vi "Goal Cases.vi"(3 "InArray":dbl[][](array[numeric])) -> (0 "Classification Error":bool, 1 "OutArray":dbl[][](array[numeric]))   [LabVIEW 2012]
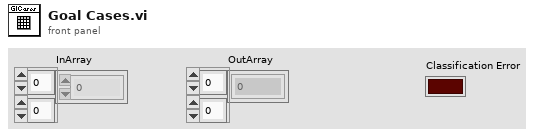
[diagram p1: front panel]
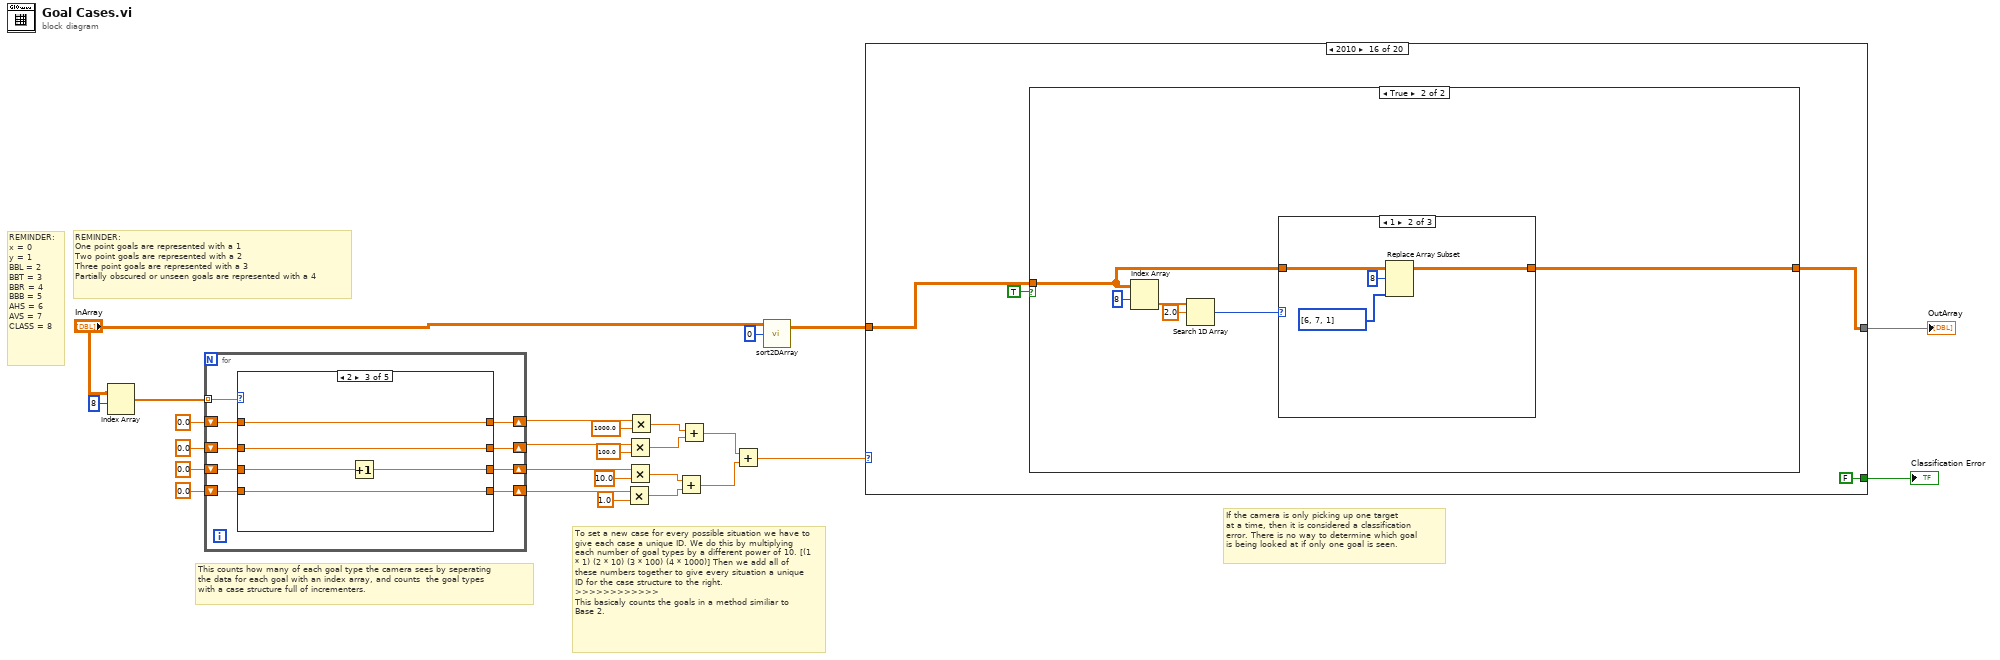
[diagram p0: block diagram]
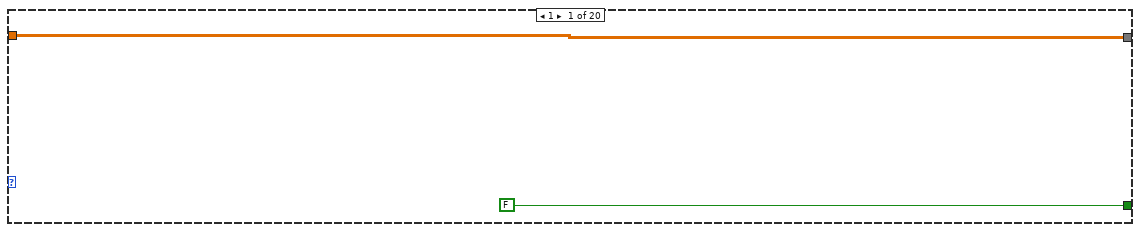
[diagram p2: hidden frame]
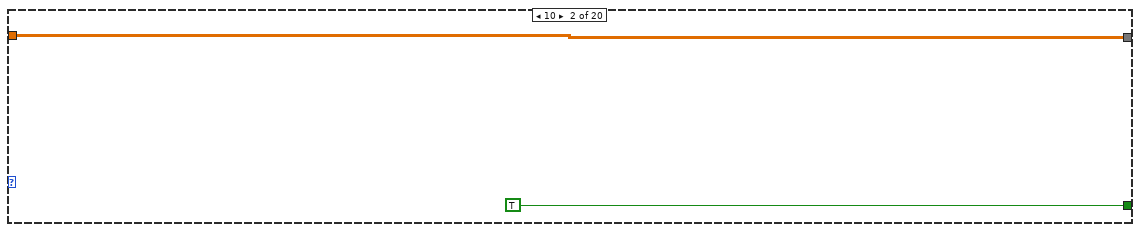
[diagram p3: hidden frame]
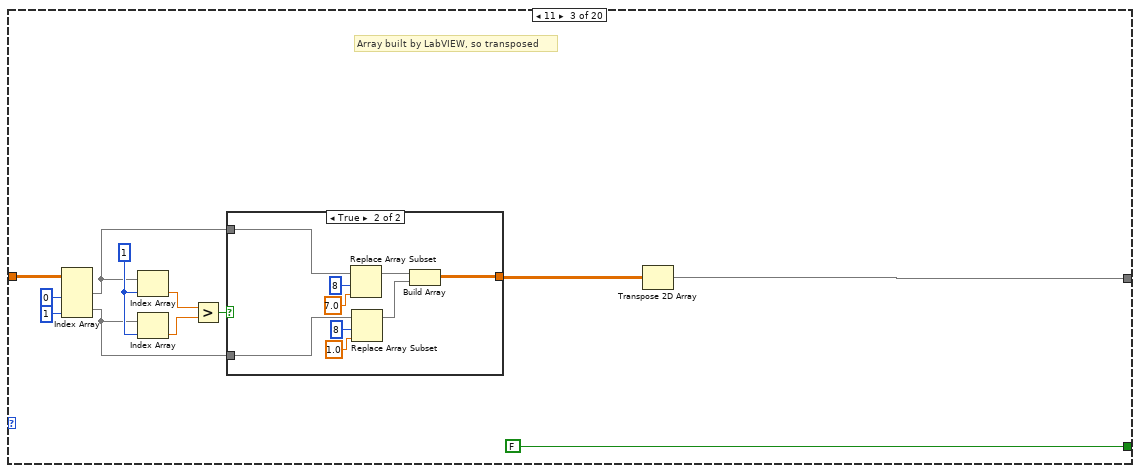
[diagram p4: hidden frame]
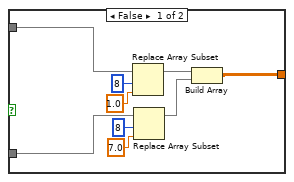
[diagram p5: hidden frame]
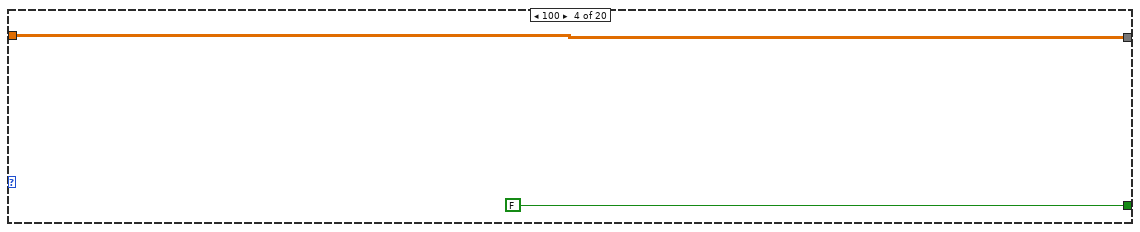
[diagram p6: hidden frame]
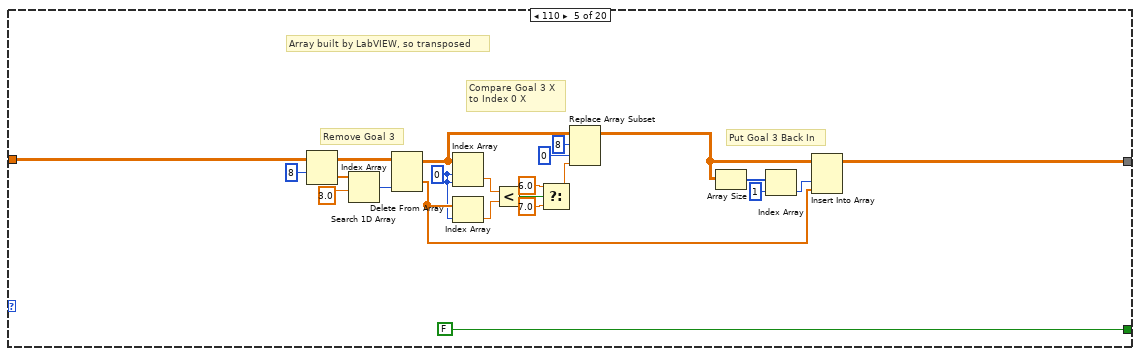
[diagram p7: hidden frame]
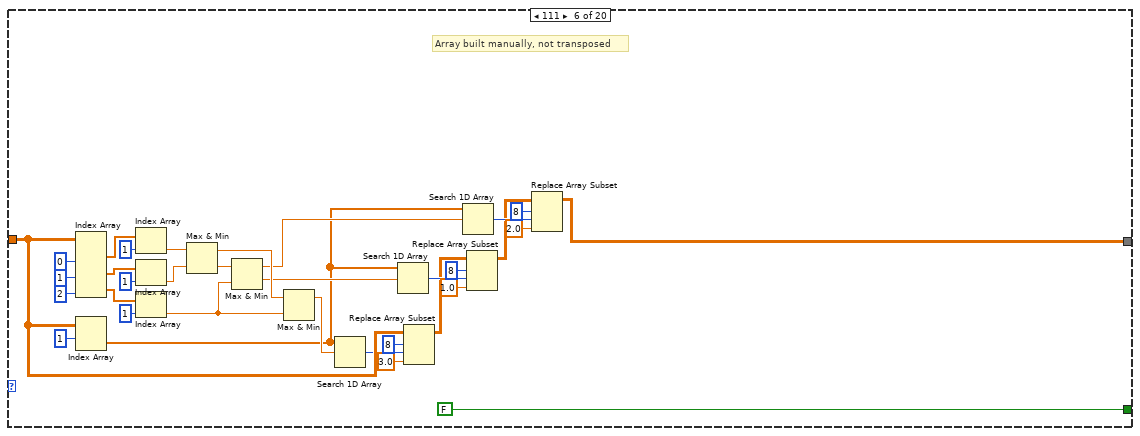
[diagram p8: hidden frame]
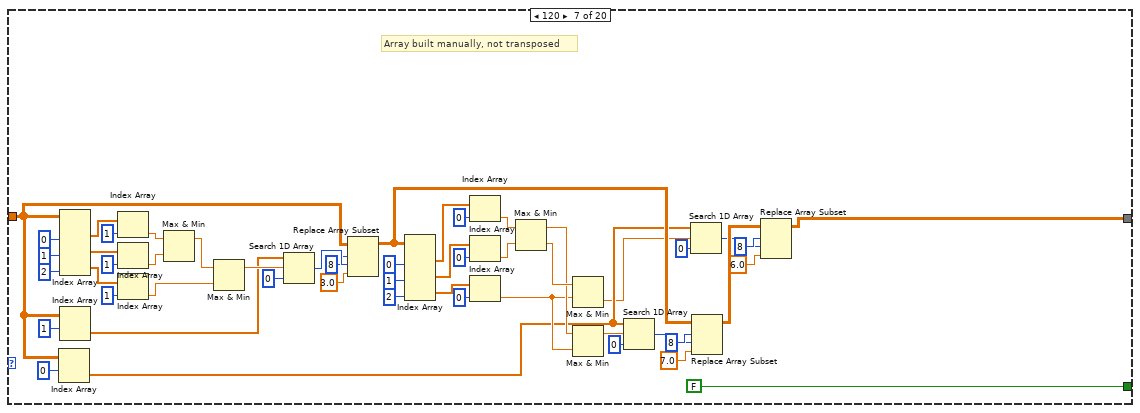
[diagram p9: hidden frame]
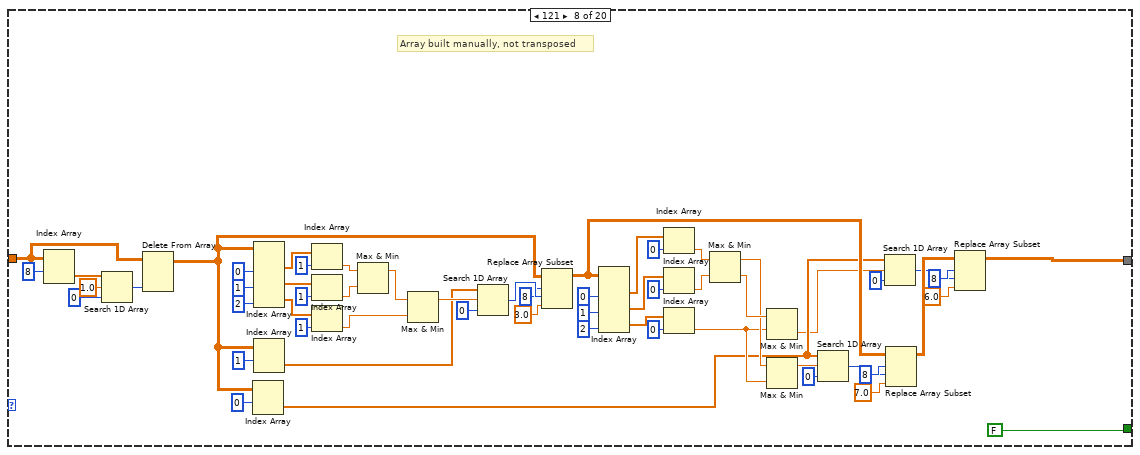
[diagram p10: hidden frame]
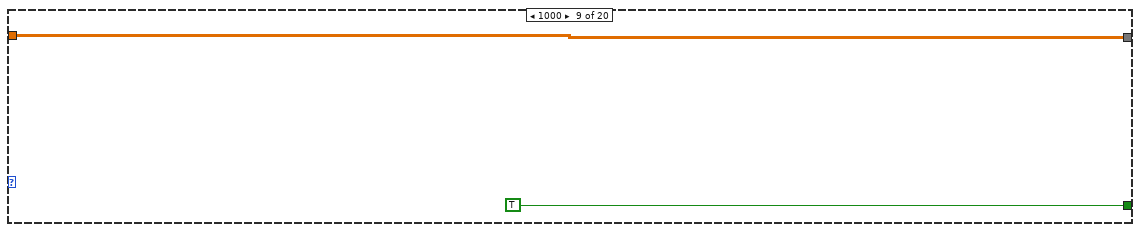
[diagram p11: hidden frame]
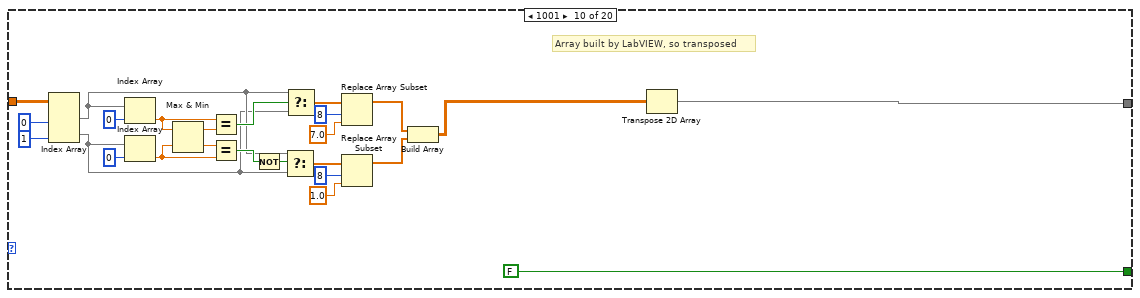
[diagram p12: hidden frame]
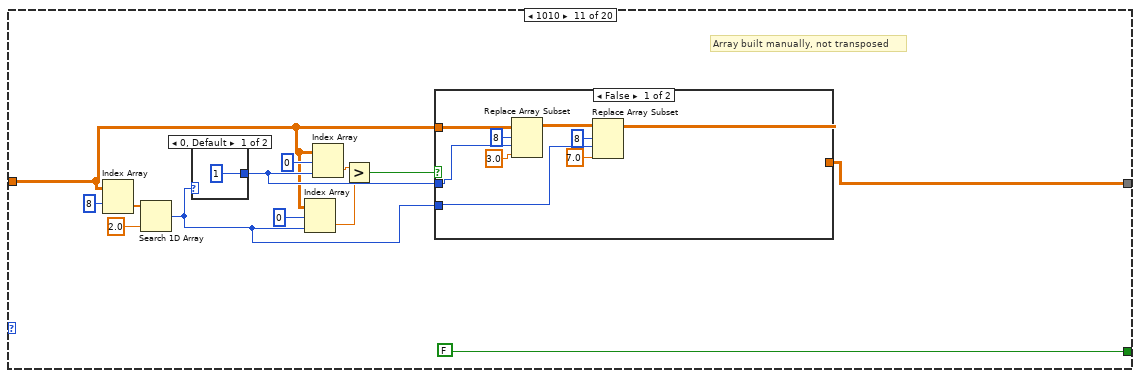
[diagram p13: hidden frame]
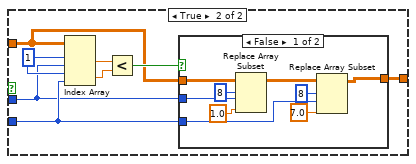
[diagram p14: hidden frame]
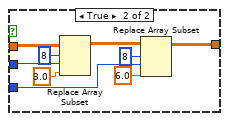
[diagram p15: hidden frame]
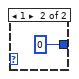
[diagram p16: hidden frame]
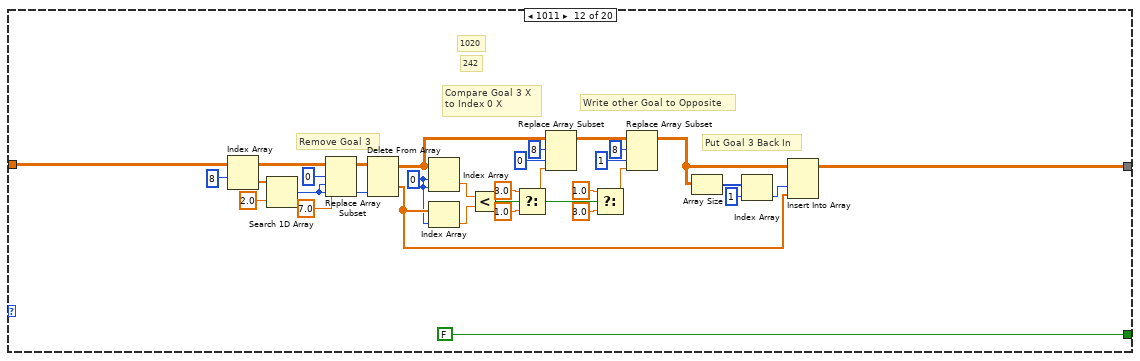
[diagram p17: hidden frame]
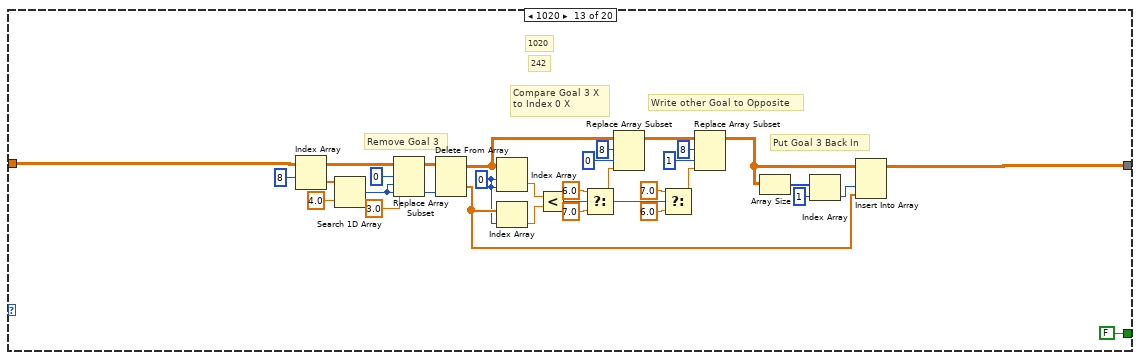
[diagram p18: hidden frame]
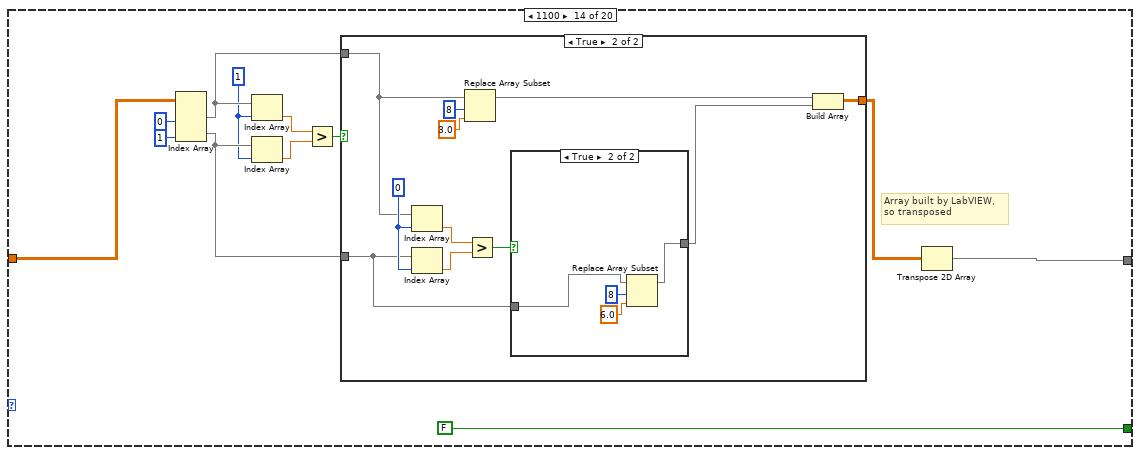
[diagram p19: hidden frame]
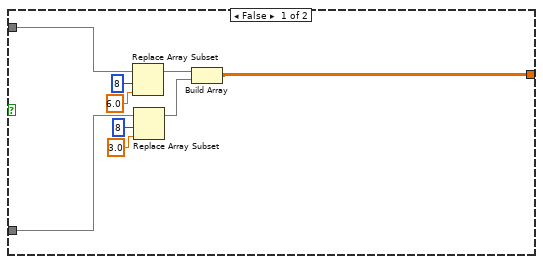
[diagram p20: hidden frame]
diagram:
  # "REMINDER:\nx = 0\ny = 1\nBBL = 2\nBBT = 3\nBBR = 4 \nBBB = 5 \nAHS = 6\nAVS = 7 \nCLASS = 8"
  # "REMINDER: \nOne point goals are represented with a 1\nTwo point goals are represented with a 2\nThree point goals are represented with a 3\nPartially obscured or unseen goals are represented with a 4"
  # "To set a new case for every possible situation we have to give each case a unique ID. We do this by multiplying each number of goal types by a different power of 10. [(1 * 1) (2 * 10) (3 * 100) (4 * 1000)] Then we add all of these numbers together to give every situation a unique ID for the case structure to the right.  >>>>>>>>>>>>\nThis basicaly counts the goals in a method similiar to Base 2."
  # "This counts how many of each goal type the camera sees by seperating\nthe data for each goal with an index array, and counts  the goal types \nwith a case structure full of incrementers."
  # "If the camera is only picking up one target\nat a time, then it is considered a classification\nerror. There is no way to determine which goal\nis being looked at if only one goal is seen."
  n1 = Index Array(array="InArray", index (row)=8) -> (element=w25:dbl[])  [unwired: 1 in]
  n2 = for {
    tunnel: w25 -> [w35] mode=indexing
    shift-right: [w34] -> w14
    shift-left: 0.0 -> [w33]
    shift-right: [w32] -> w16
    shift-left: 0.0 -> [w31]
    shift-right: [w30] -> w18
    shift-left: 0.0 -> [w29]
    shift-right: [w28] -> w20
    shift-left: 0.0 -> [w27]
    n3 = case shown="2" w35 {
      tunnel: [w39 w40 w45 w52 w59] -> w34
      tunnel: w33 -> [w39 w40 w45 w52 w58]
      tunnel: [w38 w41 w46 w54 w57] -> w32
      tunnel: w31 -> [w38 w41 w46 w53 w57]
      tunnel: [w37 w42 w49 w51 w56] -> w30
      tunnel: w29 -> [w37 w42 w48 w51 w56]
      tunnel: [w36 w44 w47 w50 w55] -> w28
      tunnel: w27 -> [w36 w43 w47 w50 w55]
      frame 0, Default {
      }
      frame 1 {
        n4 = Increment(x=w43) -> (x+1=w44:dbl)
      }
      frame 2 {
        n5 = Increment(x=w48) -> (x+1=w49:dbl)
      }
      frame 3 {
        n6 = Increment(x=w53) -> (x+1=w54:dbl)
      }
      frame 4 {
        n7 = Increment(x=w58) -> (x+1=w59:dbl)
      }
    }
  }
  n8 = Multiply(x=w20, y=1.0) -> (x*y=w12:dbl)
  n9 = Multiply(x=w16, y=100.0) -> (x*y=w9:dbl)
  n10 = Multiply(x=w18, y=10.0) -> (x*y=w11:dbl)
  n11 = Multiply(x=w14, y=1000.0) -> (x*y=w10:dbl)
  n12 = Add(x=w11, y=w12) -> (x+y=w7:dbl)
  n13 = Add(x=w10, y=w9) -> (x+y=w8:dbl)
  n14 = Add(x=w8, y=w7) -> (x+y=w4:dbl)
  n15 = call "sort2DArray.vi"("index (row)"=0, "Input Array"="InArray") -> ("Sorted Array"=w2:dbl[][])  [unwired: 3 in]
  n16 = case shown="2010" w4 {
    tunnel: [FALSE TRUE FALSE FALSE FALSE FALSE FALSE FALSE TRUE FALSE FALSE FALSE FALSE ("Boolean") FALSE FALSE FALSE ("Boolean") FALSE ("Boolean") FALSE ("Boolean") FALSE ("Boolean") TRUE ("Boolean")] -> w6
    tunnel: w2 -> [w60 w62 w74 w94 w98 w133 w174 w253 w259 w284 w287 w337 w368 w398 w438 w498 w610 w636 w669 w724]
    tunnel: [w60 w62 w64 w94 w97 w118 w153 w202 w259 w263 w286 w336 w367 w396 w439 w496 w609 w637 w668 w724] -> w5
    frame 1 {
    }
    frame 10 {
    }
    frame 11 {
      w68 = 1 ("index")
      # "Array built by LabVIEW, so transposed"
      n17 = Index Array(array=w74, index (col) #1=0 ("disabled index (col)"), index (col) #2=1 ("index (col)")) -> (element #1=w67:dbl[], element #2=w66:dbl[])  [unwired: 2 in]
      n18 = Index Array(array=w67, index=w68) -> (element=w70:dbl)
      n19 = Index Array(array=w66, index=w68) -> (element=w71:dbl)
      n20 = Greater?(x=w70, y=w71) -> (0:w69:bool)
      n21 = case shown="True" w69 {
        tunnel: [w78 w87] -> w65
        tunnel: w67 -> [w76 w85]
        tunnel: w66 -> [w77 w86]
        frame False {
          n22 = Replace Array Subset(array=w76, new element=1.0 ("new element/subarray"), index=8) -> (w80:dbl[])
          n23 = Replace Array Subset(array=w77, new element=7.0 ("new element/subarray"), index=8) -> (w79:dbl[])
          n24 = Build Array(w80, w79) -> (w78:dbl[][])
        }
        frame True {
          n25 = Replace Array Subset(array=w85, new element=7.0 ("new element/subarray"), index=8) -> (w89:dbl[])
          n26 = Replace Array Subset(array=w86, new element=1.0 ("new element/subarray"), index=8) -> (w88:dbl[])
          n27 = Build Array(w89, w88) -> (w87:dbl[][])
        }
      }
      n28 = Transpose 2D Array(2D array=w65) -> (transposed array=w64:dbl[][])
    }
    frame 100 {
    }
    frame 110 {
      w102 = 0 ("index (row)")
      # "Compare Goal 3 X\nto Index 0 X"
      # "Put Goal 3 Back In"
      # "Remove Goal 3"
      # "Array built by LabVIEW, so transposed"
      n29 = Index Array(array=w98, index (row)=8) -> (element=w115:dbl[])  [unwired: 1 in]
      n30 = Search 1D Array(1D array=w115, element=3.0) -> (index of element=w103:i32)  [unwired: 1 in]
      n31 = Delete From Array(array=w98, index (col)=w103) -> (deleted portion=w112:dbl[], array with subset deleted=w100:dbl[][])  [unwired: 2 in]
      n32 = Index Array(array=w100, index (row)=w102, index (col)=w102) -> (element=w101:dbl)
      n33 = Index Array(array=w112, index=w102) -> (element=w108:dbl)
      n34 = Less?(x=w101, y=w108) -> (x < y?=w99:bool)
      n35 = Select(t=6.0, s=w99, f=7.0) -> (s? t:f=w104:dbl)
      n36 = Replace Array Subset(array=w100, new element=w104, index (row)=8 ("disabled index (row)"), index (col)=0 ("disabled index (col)")) -> (w96:dbl[][])
      n37 = Array Size(array=w96) -> (size(s)=w111:i32[])
      n38 = Index Array(array=w111, index=1) -> (element=w109:i32)
      n39 = Insert Into Array(array=w96, index (col)=w109, new element=w112) -> (w97:dbl[][])  [unwired: 1 in]
    }
    frame 111 {
      # "Array built manually, not transposed"
      n40 = Index Array(array=w133, index (col) #1=0 ("disabled index (col)"), index (col) #2=1 ("index (col)"), index (col) #3=2 ("index (col)")) -> (element #1=w146:dbl[], element #2=w143:dbl[], element #3=w141:dbl[])  [unwired: 3 in]
      n41 = Index Array(array=w133, index (row)=1) -> (element=w119:dbl[])  [unwired: 1 in]
      n42 = Index Array(array=w146, index=1) -> (element=w140:dbl)
      n43 = Index Array(array=w143, index=1) -> (element=w139:dbl)
      n44 = Index Array(array=w141, index=1) -> (element=w136:dbl)
      n45 = Max & Min(x=w140, y=w139) -> (max(x,y)=w135:dbl, min(x,y)=w137:dbl)
      n46 = Max & Min(x=w137, y=w136) -> (max(x,y)=w120:dbl, min(x,y)=w126:dbl)
      n47 = Max & Min(x=w135, y=w136) -> (max(x,y)=w134:dbl)  [unwired: 1 out]
      n48 = Search 1D Array(1D array=w119, element=w134) -> (index of element=w132:i32)  [unwired: 1 in]
      n49 = Search 1D Array(1D array=w119, element=w126) -> (index of element=w129:i32)  [unwired: 1 in]
      n50 = Replace Array Subset(array=w133, new element=3.0 ("new element/subarray"), index (row)=8 ("disabled index (row)"), index (col)=w132) -> (w125:dbl[][])
      n51 = Search 1D Array(1D array=w119, element=w120) -> (index of element=w124:i32)  [unwired: 1 in]
      n52 = Replace Array Subset(array=w125, new element=1.0 ("new element/subarray"), index (row)=8 ("disabled index (row)"), index (col)=w129) -> (w121:dbl[][])
      n53 = Replace Array Subset(array=w121, new element=2.0 ("new element/subarray"), index (row)=8 ("disabled index (row)"), index (col)=w124) -> (w118:dbl[][])
    }
    frame 120 {
      # "Array built manually, not transposed"
      n54 = Index Array(array=w174, index (row)=0) -> (element=w161:dbl[])  [unwired: 1 in]
      n55 = Index Array(array=w174, index (col) #1=0 ("disabled index (col)"), index (col) #2=1 ("index (col)"), index (col) #3=2 ("index (col)")) -> (element #1=w197:dbl[], element #2=w193:dbl[], element #3=w192:dbl[])  [unwired: 3 in]
      n56 = Index Array(array=w174, index (row)=1) -> (element=w177:dbl[])  [unwired: 1 in]
      n57 = Index Array(array=w197, index=1) -> (element=w190:dbl)
      n58 = Index Array(array=w193, index=1) -> (element=w191:dbl)
      n59 = Index Array(array=w192, index=1) -> (element=w188:dbl)
      n60 = Max & Min(x=w190, y=w191) -> (max(x,y)=w189:dbl)  [unwired: 1 out]
      n61 = Max & Min(x=w189, y=w188) -> (max(x,y)=w187:dbl)  [unwired: 1 out]
      n62 = Search 1D Array(1D array=w177, element=w187, start index (0)=0) -> (index of element=w156:i32)
      n63 = Replace Array Subset(array=w174, new element=3.0 ("new element/subarray"), index (row)=8 ("disabled index (col)"), index (col)=w156) -> (w163:dbl[][])
      n64 = Index Array(array=w163, index (col) #1=0 ("disabled index (col)"), index (col) #2=1 ("index (col)"), index (col) #3=2 ("index (col)")) -> (element #1=w170:dbl[], element #2=w169:dbl[], element #3=w168:dbl[])  [unwired: 3 in]
      n65 = Index Array(array=w170, index=0) -> (element=w166:dbl)
      n66 = Index Array(array=w169, index=0) -> (element=w165:dbl)
      n67 = Index Array(array=w168, index=0) -> (element=w167:dbl)
      n68 = Max & Min(x=w166, y=w165) -> (max(x,y)=w179:dbl, min(x,y)=w180:dbl)
      n69 = Max & Min(x=w180, y=w167) -> (min(x,y)=w160:dbl)  [unwired: 1 out]
      n70 = Max & Min(x=w179, y=w167) -> (max(x,y)=w176:dbl)  [unwired: 1 out]
      n71 = Search 1D Array(1D array=w161, element=w176, start index (0)=0) -> (index of element=w157:i32)
      n72 = Search 1D Array(1D array=w161, element=w160, start index (0)=0) -> (index of element=w151:i32)
      n73 = Replace Array Subset(array=w163, new element=7.0 ("new element/subarray"), index (row)=8 ("disabled index (col)"), index (col)=w157) -> (w154:dbl[][])
      n74 = Replace Array Subset(array=w154, new element=6.0 ("new element/subarray"), index (row)=8 ("disabled index (col)"), index (col)=w151) -> (w153:dbl[][])
    }
    frame 121 {
      # "Array built manually, not transposed"
      n75 = Index Array(array=w253, index (row)=8 ("disabled index (col)")) -> (element=w256:dbl[])  [unwired: 1 in]
      n76 = Search 1D Array(1D array=w256, element=1.0, start index (0)=0) -> (index of element=w252:i32)
      n77 = Delete From Array(array=w253, index (col)=w252) -> (array with subset deleted=w203:dbl[][])  [unwired: 2 in, 1 out]
      n78 = Index Array(array=w203, index (row)=0) -> (element=w213:dbl[])  [unwired: 1 in]
      n79 = Index Array(array=w203, index (col) #1=0 ("disabled index (col)"), index (col) #2=1 ("index (col)"), index (col) #3=2 ("index (col)")) -> (element #1=w248:dbl[], element #2=w244:dbl[], element #3=w243:dbl[])  [unwired: 3 in]
      n80 = Index Array(array=w203, index (row)=1) -> (element=w228:dbl[])  [unwired: 1 in]
      n81 = Index Array(array=w248, index=1) -> (element=w241:dbl)
      n82 = Index Array(array=w244, index=1) -> (element=w242:dbl)
      n83 = Index Array(array=w243, index=1) -> (element=w239:dbl)
      n84 = Max & Min(x=w241, y=w242) -> (max(x,y)=w240:dbl)  [unwired: 1 out]
      n85 = Max & Min(x=w240, y=w239) -> (max(x,y)=w238:dbl)  [unwired: 1 out]
      n86 = Search 1D Array(1D array=w228, element=w238, start index (0)=0) -> (index of element=w208:i32)
      n87 = Replace Array Subset(array=w203, new element=3.0 ("new element/subarray"), index (row)=8 ("disabled index (col)"), index (col)=w208) -> (w215:dbl[][])
      n88 = Index Array(array=w215, index (col) #1=0 ("disabled index (col)"), index (col) #2=1 ("index (col)"), index (col) #3=2 ("index (col)")) -> (element #1=w222:dbl[], element #2=w221:dbl[], element #3=w220:dbl[])  [unwired: 3 in]
      n89 = Index Array(array=w222, index=0) -> (element=w218:dbl)
      n90 = Index Array(array=w221, index=0) -> (element=w217:dbl)
      n91 = Index Array(array=w220, index=0) -> (element=w219:dbl)
      n92 = Max & Min(x=w218, y=w217) -> (max(x,y)=w230:dbl, min(x,y)=w231:dbl)
      n93 = Max & Min(x=w231, y=w219) -> (min(x,y)=w212:dbl)  [unwired: 1 out]
      n94 = Max & Min(x=w230, y=w219) -> (max(x,y)=w227:dbl)  [unwired: 1 out]
      n95 = Search 1D Array(1D array=w213, element=w227, start index (0)=0) -> (index of element=w209:i32)
      n96 = Search 1D Array(1D array=w213, element=w212, start index (0)=0) -> (index of element=w204:i32)
      n97 = Replace Array Subset(array=w215, new element=7.0 ("new element/subarray"), index (row)=8 ("disabled index (col)"), index (col)=w209) -> (w206:dbl[][])
      n98 = Replace Array Subset(array=w206, new element=6.0 ("new element/subarray"), index (row)=8 ("disabled index (col)"), index (col)=w204) -> (w202:dbl[][])
    }
    frame 1000 {
    }
    frame 1001 {
      # "Array built by LabVIEW, so transposed"
      n99 = Index Array(array=w284, index (col) #1=0 ("index (row)"), index (col) #2=1 ("index (row)")) -> (element #1=w271:dbl[], element #2=w270:dbl[])  [unwired: 2 in]
      n100 = Index Array(array=w271, index=0) -> (element=w275:dbl)
      n101 = Index Array(array=w270, index=0) -> (element=w277:dbl)
      n102 = Max & Min(x=w275, y=w277) -> (max(x,y)=w276:dbl, min(x,y)=w278:dbl)
      n103 = Equal?(x=w275, y=w276) -> (x = y?=w272:bool)
      n104 = Equal?(x=w278, y=w277) -> (x = y?=w273:bool)
      n105 = Not(x=w273) -> (.not. x?=w274:bool)
      n106 = Select(t=w271, s=w274, f=w270) -> (s? t:f=w281:dbl[])
      n107 = Select(t=w271, s=w272, f=w270) -> (s? t:f=w267:dbl[])
      n108 = Replace Array Subset(array=w267, new element=7.0 ("new element/subarray"), index=8) -> (w266:dbl[])
      n109 = Replace Array Subset(array=w281, new element=1.0 ("new element/subarray"), index=8) -> (w265:dbl[])
      n110 = Build Array(w266, w265) -> (w264:dbl[][])
      n111 = Transpose 2D Array(2D array=w264) -> (transposed array=w263:dbl[][])
    }
    frame 1010 {
      # "Array built manually, not transposed"
      n112 = Index Array(array=w287, index (row)=8 ("index")) -> (element=w289:dbl[])  [unwired: 1 in]
      n113 = Search 1D Array(1D array=w289, element=2.0) -> (index of element=w297:i32)  [unwired: 1 in]
      n114 = case shown="0, Default" w297 {
        tunnel: [1 0] -> w296
        frame 0, Default {
        }
        frame 1 {
        }
      }
      n115 = Index Array(array=w287, index (row)=0 ("disabled index (row)"), index (col)=w297) -> (element=w294:dbl)
      n116 = Index Array(array=w287, index (row)=0 ("disabled index (row)"), index (col)=w296) -> (element=w293:dbl)
      n117 = Greater?(x=w293, y=w294) -> (0:w295:bool)
      n118 = case shown="False" w295 {
        tunnel: w287 -> [w307 w311]
        tunnel: w296 -> [w305 w309]
        tunnel: w297 -> [w301 w310]
        tunnel: [w299 w308] -> w286
        frame False {
          n119 = Replace Array Subset(array=w307, new element=3.0 ("new element/subarray"), index (row)=8, index (col)=w305) -> (w303:dbl[][])
          n120 = Replace Array Subset(array=w303, new element=7.0 ("new element/subarray"), index (row)=8, index (col)=w301) -> (w299:dbl[][])
        }
        frame True {
          w315 = 1 ("index (row)")
          n121 = Index Array(array=w311, index (row) #1=w315, index (col) #1=w309, index (row) #2=w315, index (col) #2=w310) -> (element #1=w314:dbl, element #2=w313:dbl)
          n122 = Less?(x=w314, y=w313) -> (x < y?=w312:bool)
          n123 = case shown="False" w312 {
            tunnel: w311 -> [w319 w328]
            tunnel: w310 -> [w317 w327]
            tunnel: w309 -> [w318 w326]
            tunnel: [w316 w325] -> w308
            frame False {
              n124 = Replace Array Subset(array=w319, new element=1.0 ("new element/subarray"), index (row)=8, index (col)=w318) -> (w322:dbl[][])
              n125 = Replace Array Subset(array=w322, new element=7.0 ("new element/subarray"), index (row)=8, index (col)=w317) -> (w316:dbl[][])
            }
            frame True {
              n126 = Replace Array Subset(array=w328, new element=3.0 ("new element/subarray"), index (row)=8, index (col)=w326) -> (w331:dbl[][])
              n127 = Replace Array Subset(array=w331, new element=6.0 ("new element/subarray"), index (row)=8, index (col)=w327) -> (w325:dbl[][])
            }
          }
        }
      }
    }
    frame 1011 {
      w351 = 0 ("index (row)")
      # "Write other Goal to Opposite"
      # "Compare Goal 3 X\nto Index 0 X"
      # "Put Goal 3 Back In"
      # "Remove Goal 3"
      # "242"
      # "1020"
      n128 = Index Array(array=w337, index (row)=8) -> (element=w363:dbl[])  [unwired: 1 in]
      n129 = Search 1D Array(1D array=w363, element=2.0) -> (index of element=w340:i32)  [unwired: 1 in]
      n130 = Replace Array Subset(array=w337, new element=7.0 ("new element/subarray"), index (row)=0 ("disabled index (row)"), index (col)=w340) -> (w341:dbl[][])
      n131 = Delete From Array(array=w341, index (col)=w340) -> (deleted portion=w360:dbl[], array with subset deleted=w347:dbl[][])  [unwired: 2 in]
      n132 = Index Array(array=w347, index (row)=w351, index (col)=w351) -> (element=w350:dbl)
      n133 = Index Array(array=w360, index=w351) -> (element=w356:dbl)
      n134 = Less?(x=w350, y=w356) -> (x < y?=w344:bool)
      n135 = Select(t=3.0, s=w344, f=1.0) -> (s? t:f=w352:dbl)
      n136 = Replace Array Subset(array=w347, new element=w352, index (row)=8 ("disabled index (row)"), index (col)=0 ("disabled index (col)")) -> ()  [unwired: 1 out]
      n137 = Select(t=1.0, s=w344, f=3.0) -> (s? t:f=w343:dbl)
      n138 = Replace Array Subset(array=w347, new element=w343, index (row)=8 ("disabled index (row)"), index (col)=1 ("disabled index (col)")) -> (w342:dbl[][])
      n139 = Array Size(array=w342) -> (size(s)=w359:i32[])
      n140 = Index Array(array=w359, index=1) -> (element=w357:i32)
      n141 = Insert Into Array(array=w342, index (col)=w357, new element=w360) -> (w336:dbl[][])  [unwired: 1 in]
    }
    frame 1020 {
      w382 = 0 ("index (row)")
      # "Write other Goal to Opposite"
      # "Compare Goal 3 X\nto Index 0 X"
      # "Put Goal 3 Back In"
      # "Remove Goal 3"
      # "242"
      # "1020"
      n142 = Index Array(array=w368, index (row)=8) -> (element=w394:dbl[])  [unwired: 1 in]
      n143 = Search 1D Array(1D array=w394, element=4.0) -> (index of element=w371:i32)  [unwired: 1 in]
      n144 = Replace Array Subset(array=w368, new element=3.0 ("new element/subarray"), index (row)=0 ("disabled index (row)"), index (col)=w371) -> (w372:dbl[][])
      n145 = Delete From Array(array=w372, index (col)=w371) -> (deleted portion=w391:dbl[], array with subset deleted=w378:dbl[][])  [unwired: 2 in]
      n146 = Index Array(array=w378, index (row)=w382, index (col)=w382) -> (element=w381:dbl)
      n147 = Index Array(array=w391, index=w382) -> (element=w387:dbl)
      n148 = Less?(x=w381, y=w387) -> (x < y?=w375:bool)
      n149 = Select(t=6.0, s=w375, f=7.0) -> (s? t:f=w383:dbl)
      n150 = Replace Array Subset(array=w378, new element=w383, index (row)=8 ("disabled index (row)"), index (col)=0 ("disabled index (col)")) -> ()  [unwired: 1 out]
      n151 = Select(t=7.0, s=w375, f=6.0) -> (s? t:f=w374:dbl)
      n152 = Replace Array Subset(array=w378, new element=w374, index (row)=8 ("disabled index (row)"), index (col)=1 ("disabled index (col)")) -> (w373:dbl[][])
      n153 = Array Size(array=w373) -> (size(s)=w390:i32[])
      n154 = Index Array(array=w390, index=1) -> (element=w388:i32)
      n155 = Insert Into Array(array=w373, index (col)=w388, new element=w391) -> (w367:dbl[][])  [unwired: 1 in]
    }
    frame 1100 {
      w404 = 1 ("index")
      # "Array built by LabVIEW,\nso transposed"
      n156 = Index Array(array=w398, index (col) #1=0 ("disabled index (col)"), index (col) #2=1 ("index (col)")) -> (element #1=w405:dbl[], element #2=w406:dbl[])  [unwired: 2 in]
      n157 = Index Array(array=w405, index=w404) -> (element=w402:dbl)
      n158 = Index Array(array=w406, index=w404) -> (element=w401:dbl)
      n159 = Greater?(x=w402, y=w401) -> (0:w403:bool)
      n160 = case shown="True" w403 {
        tunnel: [w410 w424] -> w397
        tunnel: w405 -> [w408 w419]
        tunnel: w406 -> [w409 w418]
        frame False {
          n161 = Replace Array Subset(array=w408, new element=6.0 ("new element/subarray"), index=8) -> (w412:dbl[])
          n162 = Replace Array Subset(array=w409, new element=3.0 ("new element/subarray"), index=8) -> (w411:dbl[])
          n163 = Build Array(w412, w411) -> (w410:dbl[][])
        }
        frame True {
          w421 = 0 ("index")
          n164 = Index Array(array=w419, index=w421) -> (element=w422:dbl)
          n165 = Index Array(array=w418, index=w421) -> (element=w423:dbl)
          n166 = Replace Array Subset(array=w419, new element=3.0 ("new element/subarray"), index=8) -> (w425:dbl[])
          n167 = Greater?(x=w422, y=w423) -> (0:w420:bool)
          n168 = case shown="True" w420 {
            tunnel: w418 -> [w429 w433]
            tunnel: [w428 w432] -> w417
            frame False {
              n169 = Replace Array Subset(array=w429, new element=7.0 ("new element/subarray"), index=8) -> (w428:dbl[])
            }
            frame True {
              n170 = Replace Array Subset(array=w433, new element=6.0 ("new element/subarray"), index=8) -> (w432:dbl[])
            }
          }
          n171 = Build Array(w425, w417) -> (w424:dbl[][])
        }
      }
      n172 = Transpose 2D Array(2D array=w397) -> (transposed array=w396:dbl[][])
    }
    frame 1110 {
      # "Array built by LabVIEW,\nso transposed"
      # "Goal 2, 3, Then 4 Subarrays"
      n173 = Transpose 2D Array(2D array=w438) -> (transposed array=w437:dbl[][])
      n174 = Index Array(array=w437, index (col)=8 ("disabled index (col)")) -> (element=w451:dbl[])  [unwired: 1 in]
      n175 = Search 1D Array(1D array=w451, element=2.0) -> (index of element=w436:i32)  [unwired: 1 in]
      n176 = Search 1D Array(1D array=w451, element=3.0) -> (index of element=w450:i32)  [unwired: 1 in]
      n177 = Search 1D Array(1D array=w451, element=4.0) -> (index of element=w449:i32)  [unwired: 1 in]
      n178 = Index Array(array=w437, index (row)=w436) -> (element=w443:dbl[])  [unwired: 1 in]
      n179 = Index Array(array=w437, index (row)=w450) -> (element=w442:dbl[])  [unwired: 1 in]
      n180 = Index Array(array=w437, index (row)=w449) -> (element=w441:dbl[])  [unwired: 1 in]
      n181 = Index Array(array=w443, index=0) -> (element=w447:dbl)
      n182 = Index Array(array=w442, index=0) -> (element=w448:dbl)
      n183 = Greater?(x=w447, y=w448) -> (0:w446:bool)
      n184 = case shown="True" w446 {
        tunnel: w443 -> [w459 w490]
        tunnel: w442 -> [w460 w489]
        tunnel: w441 -> [w458 w495]
        tunnel: [w457 w486] -> w440
        frame False {
          n185 = Index Array(array=w459, index=0) -> (element=w462:dbl)
          n186 = Index Array(array=w458, index=0) -> (element=w463:dbl)
          n187 = Greater?(x=w462, y=w463) -> (0:w461:bool)
          n188 = case shown="False" w461 {
            tunnel: w460 -> [w469 w479]
            tunnel: w459 -> [w468 w478]
            tunnel: w458 -> [w467 w477]
            tunnel: [w466 w476] -> w457
            frame False {
              n189 = Replace Array Subset(array=w468, new element=6.0 ("new element/subarray"), index=8) -> (w471:dbl[])
              n190 = Replace Array Subset(array=w467, new element=7.0 ("new element/subarray"), index=8) -> (w470:dbl[])
              n191 = Build Array(w471, w469, w470) -> (w466:dbl[][])
            }
            frame True {
              n192 = Replace Array Subset(array=w478, new element=7.0 ("new element/subarray"), index=8) -> (w481:dbl[])
              n193 = Replace Array Subset(array=w477, new element=1.0 ("new element/subarray"), index=8) -> (w480:dbl[])
              n194 = Build Array(w481, w479, w480) -> (w476:dbl[][])
            }
          }
        }
        frame True {
          n195 = Replace Array Subset(array=w490, new element=7.0 ("new element/subarray"), index=8) -> (w488:dbl[])
          n196 = Replace Array Subset(array=w495, new element=6.0 ("new element/subarray"), index=8) -> (w487:dbl[])
          n197 = Build Array(w488, w489, w487) -> (w486:dbl[][])
        }
      }
      n198 = Transpose 2D Array(2D array=w440) -> (transposed array=w439:dbl[][])
    }
    frame 2010 {
      n199 = case shown="True" TRUE {
        tunnel: w498 -> [w501 w590]
        tunnel: [w500 w591] -> w496
        frame False {
          w519 = 0 ("index (row)")
          w526 = 0 ("index (row)")
          w527 = 8 ("index (row)")
          # "If both 4s are greater than 2, it's a 1\nIf both 4s are less than 2, it's a 2\nIf niether, it's a 0"
          # "Index 1 X"
          # "Index 0 X"
          # "0 is 424\n1 is 244\n2 is 442"
          # "244"
          # "Put Goal 3 Back In"
          # "Rename 2 to 7 and remove"
          # "442"
          # "424"
          # "2010"
          n200 = Index Array(array=w501, index (row)=w527) -> (element=w535:dbl[])  [unwired: 1 in]
          n201 = Search 1D Array(1D array=w535, element=2.0) -> (index of element=w529:i32)  [unwired: 1 in]
          n202 = Replace Array Subset(array=w501, new element=7.0 ("new element/subarray"), index (row)=w527, index (col)=w529) -> (w530:dbl[][])
          n203 = Delete From Array(array=w530, index (col)=w529) -> (deleted portion=w504:dbl[], array with subset deleted=w505:dbl[][])  [unwired: 2 in]
          n204 = Index Array(array=w505, index (row)=w526, index (col)=w526) -> (element=w507:dbl)
          n205 = Index Array(array=w504, index=w526) -> (element=w524:dbl)
          n206 = Index Array(array=w505, index (row)=w526, index (col)=1 ("disabled index (col)")) -> (element=w506:dbl)
          n207 = Index Array(array=w505, index (row)=w519, index (col)=w519) -> (element=w523:dbl)
          n208 = Index Array(array=w504, index=w519) -> (element=w520:dbl)
          n209 = Index Array(array=w505, index (row)=w519, index (col)=1 ("disabled index (col)")) -> (element=w521:dbl)
          n210 = Less?(x=w507, y=w524) -> (x < y?=w517:bool)
          n211 = Greater?(x=w524, y=w506) -> (0:w518:bool)
          n212 = Greater?(x=w523, y=w520) -> (0:w516:bool)
          n213 = Less?(x=w520, y=w521) -> (x < y?=w515:bool)
          n214 = And(x=w517, y=w518) -> (x .and. y?=w512:bool)
          n215 = And(x=w516, y=w515) -> (x .and. y?=w514:bool)
          n216 = Select(t=1, s=w514, f=0) -> (s? t:f=w511:i32)
          n217 = Select(t=2, s=w512, f=w511) -> (s? t:f=w508:i32)
          n218 = case shown="1" w508 {
            tunnel: w507 -> [w552 w572 w589]
            tunnel: w506 -> [w551 w571 w588]
            tunnel: w505 -> [w541 w561 w578]
            tunnel: [w537 w557 w574] -> w502
            tunnel: w504 -> [w536 w556 w573]
            tunnel: [w536 w553 w573] -> w503
            frame 0, Default {
              # "2 is 7, leave as 7"
              n219 = Greater?(x=w552, y=w551) -> (0:w542:bool)
              n220 = Select(t=7.0, s=w542, f=6.0) -> (s? t:f=w547:dbl)
              n221 = Replace Array Subset(array=w541, new element=w547, index (row)=8 ("disabled index (row)"), index (col)=0 ("disabled index (col)")) -> (w538:dbl[][])
              n222 = Select(t=6.0, s=w542, f=7.0) -> (s? t:f=w543:dbl)
              n223 = Replace Array Subset(array=w538, new element=w543, index (row)=8 ("disabled index (row)"), index (col)=1 ("disabled index (col)")) -> (w537:dbl[][])
            }
            frame 1 {
              # "2 is 6, change to 6"
              n224 = Greater?(x=w572, y=w571) -> (0:w562:bool)
              n225 = Select(t=7.0, s=w562, f=3.0) -> (s? t:f=w567:dbl)
              n226 = Replace Array Subset(array=w561, new element=w567, index (row)=8 ("disabled index (row)"), index (col)=0 ("disabled index (col)")) -> (w558:dbl[][])
              n227 = Select(t=3.0, s=w562, f=7.0) -> (s? t:f=w563:dbl)
              n228 = Replace Array Subset(array=w556, new element=6.0 ("new element/subarray"), index=8) -> (w553:dbl[])
              n229 = Replace Array Subset(array=w558, new element=w563, index (row)=8 ("disabled index (row)"), index (col)=1 ("disabled index (col)")) -> (w557:dbl[][])
            }
            frame 2 {
              # "2 is 7, leave as 7"
              n230 = Greater?(x=w589, y=w588) -> (0:w579:bool)
              n231 = Select(t=3.0, s=w579, f=6.0) -> (s? t:f=w584:dbl)
              n232 = Replace Array Subset(array=w578, new element=w584, index (row)=8 ("disabled index (row)"), index (col)=0 ("disabled index (col)")) -> (w575:dbl[][])
              n233 = Select(t=6.0, s=w579, f=3.0) -> (s? t:f=w580:dbl)
              n234 = Replace Array Subset(array=w575, new element=w580, index (row)=8 ("disabled index (row)"), index (col)=1 ("disabled index (col)")) -> (w574:dbl[][])
            }
          }
          n235 = Array Size(array=w502) -> (size(s)=w533:i32[])
          n236 = Index Array(array=w533, index=1) -> (element=w531:i32)
          n237 = Insert Into Array(array=w502, index (col)=w531, new element=w503) -> (w500:dbl[][])  [unwired: 1 in]
        }
        frame True {
          n238 = Index Array(array=w590, index (row)=8) -> (element=w594:dbl[])  [unwired: 1 in]
          n239 = Search 1D Array(1D array=w594, element=2.0) -> (index of element=w592:i32)  [unwired: 1 in]
          n240 = case shown="1" w592 {
            tunnel: w590 -> [w599 w603 w607]
            tunnel: [w596 w600 w604] -> w591
            frame 0, Default {
              n241 = Replace Array Subset(array=w599, new element=i32[] [6, 3, 7], index (row)=8) -> (w596:dbl[][])  [unwired: 1 in]
            }
            frame 1 {
              # "3"
              n242 = Replace Array Subset(array=w603, new element=i32[] [6, 7, 1], index (row)=8) -> (w600:dbl[][])  [unwired: 1 in]
            }
            frame 2 {
              n243 = Replace Array Subset(array=w607, new element=i32[] [6, 3, 7], index (row)=8) -> (w604:dbl[][])  [unwired: 1 in]
            }
          }
        }
      }
    }
    frame 2100 {
      w620 = 0 ("index (row)")
      # "Write other Goal to Opposite"
      # "Compare Goal 3 X\nto Index 0 X"
      # "Put Goal 3 Back In"
      # "Remove Goal 3"
      n244 = Index Array(array=w610, index (row)=8) -> (element=w633:dbl[])  [unwired: 1 in]
      n245 = Search 1D Array(1D array=w633, element=3.0) -> (index of element=w621:i32)  [unwired: 1 in]
      n246 = Delete From Array(array=w610, index (col)=w621) -> (deleted portion=w630:dbl[], array with subset deleted=w616:dbl[][])  [unwired: 2 in]
      n247 = Index Array(array=w616, index (row)=w620, index (col)=w620) -> (element=w619:dbl)
      n248 = Index Array(array=w630, index=w620) -> (element=w626:dbl)
      n249 = Less?(x=w619, y=w626) -> (x < y?=w613:bool)
      n250 = Select(t=6.0, s=w613, f=7.0) -> (s? t:f=w622:dbl)
      n251 = Replace Array Subset(array=w616, new element=w622, index (row)=8 ("disabled index (row)"), index (col)=0 ("disabled index (col)")) -> ()  [unwired: 1 out]
      n252 = Select(t=7.0, s=w613, f=6.0) -> (s? t:f=w612:dbl)
      n253 = Replace Array Subset(array=w616, new element=w612, index (row)=8 ("disabled index (row)"), index (col)=1 ("disabled index (col)")) -> (w611:dbl[][])
      n254 = Array Size(array=w611) -> (size(s)=w629:i32[])
      n255 = Index Array(array=w629, index=1) -> (element=w627:i32)
      n256 = Insert Into Array(array=w611, index (col)=w627, new element=w630) -> (w609:dbl[][])  [unwired: 1 in]
    }
    frame 2110 {
      w646 = 8 ("index (row)")
      w650 = 8 ("index (row)")
      w658 = 0 ("index (row)")
      # "Put Goal 3 Back In"
      # "Compare Goal 3 X to all\nother X to find the one thats\nfarthest to the right"
      # "Remove Goal 3"
      # "Make Right 4 Goal 1"
      # "Make Goal 2 Goal 7"
      # "4324"
      # "4432"
      # "2110"
      n257 = Index Array(array=w636, index (row)=8) -> (element=w661:dbl[])  [unwired: 1 in]
      n258 = Search 1D Array(1D array=w661, element=3.0) -> (index of element=w638:i32)  [unwired: 1 in]
      n259 = Delete From Array(array=w636, index (col)=w638) -> (deleted portion=w643:dbl[], array with subset deleted=w642:dbl[][])  [unwired: 2 in]
      n260 = Index Array(array=w642, index (row)=w658) -> (element=w660:dbl[])  [unwired: 1 in]
      n261 = Index Array(array=w643, index=w658) -> (element=w657:dbl)
      n262 = for {
        tunnel: w660 -> [w665] mode=indexing
        tunnel: w657 -> [w666]
        tunnel: [w665] -> _ mode=indexing if=w663
        tunnel: [w664] -> w654 if=w663
        i -> [w664]
        n263 = Less?(x=w665, y=w666) -> (x < y?=w663:bool)
      }
      n264 = Replace Array Subset(array=w642, new element=0.0 ("new element/subarray"), index (row)=8 ("disabled index (row)"), index (col)=w654) -> ()  [unwired: 1 out]
      n265 = Index Array(array=w642, index (row)=w650) -> (element=w653:dbl[])  [unwired: 1 in]
      n266 = Search 1D Array(1D array=w653, element=2.0) -> (index of element=w651:i32)  [unwired: 1 in]
      n267 = Replace Array Subset(array=w642, new element=7.0 ("new element/subarray"), index (row)=w650, index (col)=w651) -> ()  [unwired: 1 out]
      n268 = Index Array(array=w642, index (row)=w646) -> (element=w649:dbl[])  [unwired: 1 in]
      n269 = Search 1D Array(1D array=w649, element=4.0) -> (index of element=w647:i32)  [unwired: 1 in]
      n270 = Replace Array Subset(array=w642, new element=1.0 ("new element/subarray"), index (row)=w646, index (col)=w647) -> ()  [unwired: 1 out]
      n271 = Array Size(array=w642) -> (size(s)=w641:i32[])
      n272 = Index Array(array=w641, index=1) -> (element=w639:i32)
      n273 = Insert Into Array(array=w642, index (col)=w639, new element=w643) -> (w637:dbl[][])  [unwired: 1 in]
    }
    frame 2120 {
      # "Array built manually, not transposed"
      n274 = Index Array(array=w669, index (row)=8 ("disabled index (col)")) -> (element=w722:dbl[])  [unwired: 1 in]
      n275 = Search 1D Array(1D array=w722, element=4.0, start index (0)=0) -> (index of element=w719:i32)
      n276 = Delete From Array(array=w669, index (col)=w719) -> (array with subset deleted=w670:dbl[][])  [unwired: 2 in, 1 out]
      n277 = Index Array(array=w670, index (row)=0) -> (element=w680:dbl[])  [unwired: 1 in]
      n278 = Index Array(array=w670, index (col) #1=0 ("disabled index (col)"), index (col) #2=1 ("index (col)"), index (col) #3=2 ("index (col)")) -> (element #1=w715:dbl[], element #2=w711:dbl[], element #3=w710:dbl[])  [unwired: 3 in]
      n279 = Index Array(array=w670, index (row)=1) -> (element=w695:dbl[])  [unwired: 1 in]
      n280 = Index Array(array=w715, index=1) -> (element=w708:dbl)
      n281 = Index Array(array=w711, index=1) -> (element=w709:dbl)
      n282 = Index Array(array=w710, index=1) -> (element=w706:dbl)
      n283 = Max & Min(x=w708, y=w709) -> (max(x,y)=w707:dbl)  [unwired: 1 out]
      n284 = Max & Min(x=w707, y=w706) -> (max(x,y)=w705:dbl)  [unwired: 1 out]
      n285 = Search 1D Array(1D array=w695, element=w705, start index (0)=0) -> (index of element=w675:i32)
      n286 = Replace Array Subset(array=w670, new element=3.0 ("new element/subarray"), index (row)=8 ("disabled index (col)"), index (col)=w675) -> (w682:dbl[][])
      n287 = Index Array(array=w682, index (col) #1=0 ("disabled index (col)"), index (col) #2=1 ("index (col)"), index (col) #3=2 ("index (col)")) -> (element #1=w689:dbl[], element #2=w688:dbl[], element #3=w687:dbl[])  [unwired: 3 in]
      n288 = Index Array(array=w689, index=0) -> (element=w685:dbl)
      n289 = Index Array(array=w688, index=0) -> (element=w684:dbl)
      n290 = Index Array(array=w687, index=0) -> (element=w686:dbl)
      n291 = Max & Min(x=w685, y=w684) -> (max(x,y)=w697:dbl, min(x,y)=w698:dbl)
      n292 = Max & Min(x=w698, y=w686) -> (min(x,y)=w679:dbl)  [unwired: 1 out]
      n293 = Max & Min(x=w697, y=w686) -> (max(x,y)=w694:dbl)  [unwired: 1 out]
      n294 = Search 1D Array(1D array=w680, element=w694, start index (0)=0) -> (index of element=w676:i32)
      n295 = Search 1D Array(1D array=w680, element=w679, start index (0)=0) -> (index of element=w671:i32)
      n296 = Replace Array Subset(array=w682, new element=7.0 ("new element/subarray"), index (row)=8 ("disabled index (col)"), index (col)=w676) -> (w673:dbl[][])
      n297 = Replace Array Subset(array=w673, new element=6.0 ("new element/subarray"), index (row)=8 ("disabled index (col)"), index (col)=w671) -> (w668:dbl[][])
    }
    frame 9999, Default {
    }
  }
  "OutArray" <- w5
  "Classification Error" <- w6
